vi "Queue_Driver.vi"(0 "Data_In":string, 1 "Max_Queue_Size (-1, unlimited)":i32=-1, 2 "Queue_Name":string, 5 "Data_In_N":string[](array[string]), 7 "Timeout (-1)":i32, 11 "Error_In":errorcluster, 13 "Queue_Operation_Select":T1=enum."Release_Queue") -> (4 "Data_Out":string, 15 "Error_Out":errorcluster)   [LabVIEW 2021]
doc: "This is the queue driver vi that creates, enqueues, dequeues and releases the queue."
uses:
  Control/Queue_Operation_Select.ctl
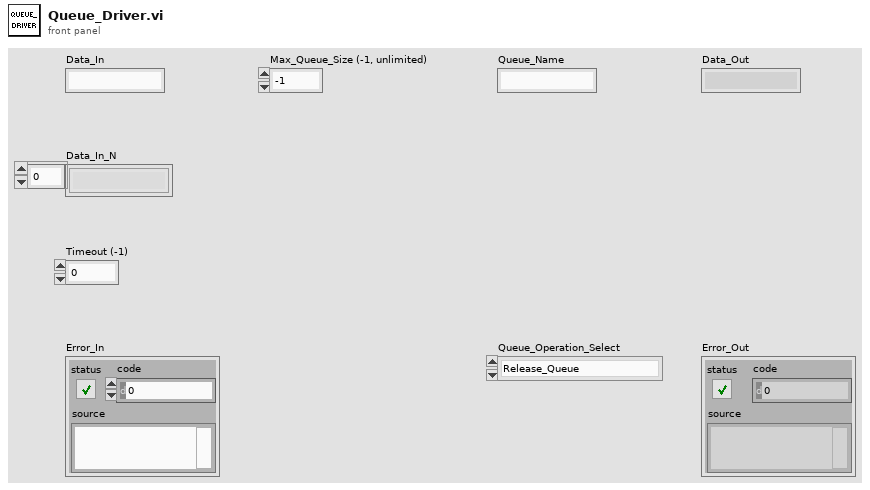
[diagram p1: front panel]
types:
  T1 = typedef "Queue_Operation_Select.ctl" = enum16{"Obtain_Queue", "Enqueue", "Enqueue_N", "Enqueue_at_First", "Dequeue", "Flush_Queue", "Release_Queue"}
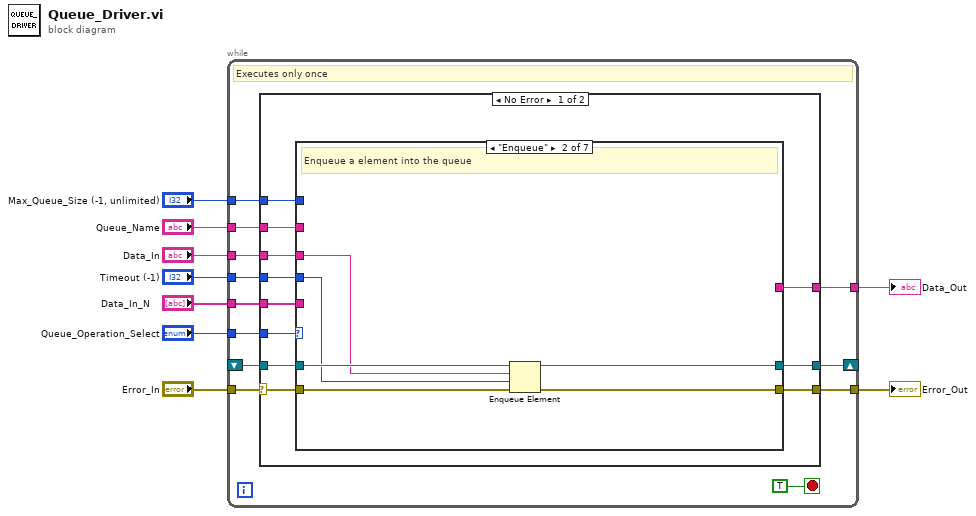
[diagram p0: block diagram]
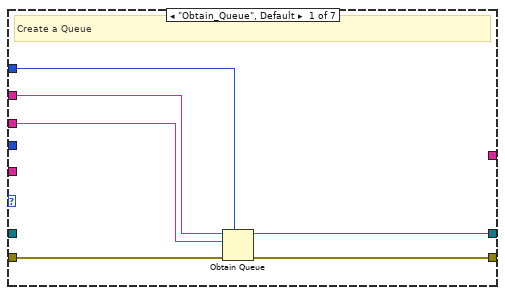
[diagram p2: hidden frame]
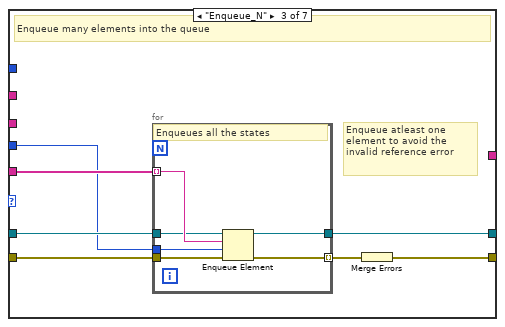
[diagram p3: hidden frame]
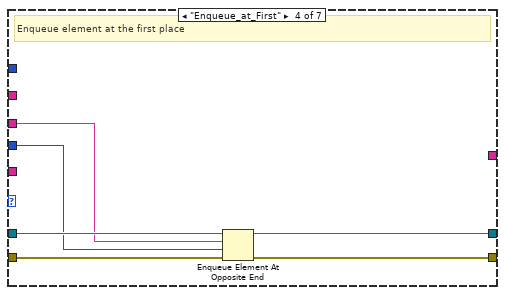
[diagram p4: hidden frame]
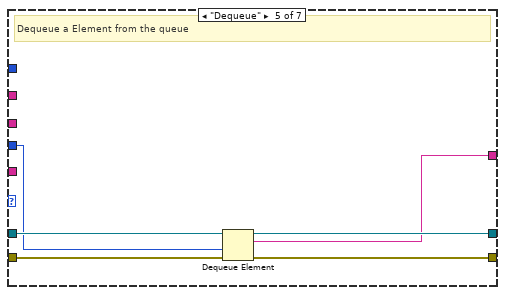
[diagram p5: hidden frame]
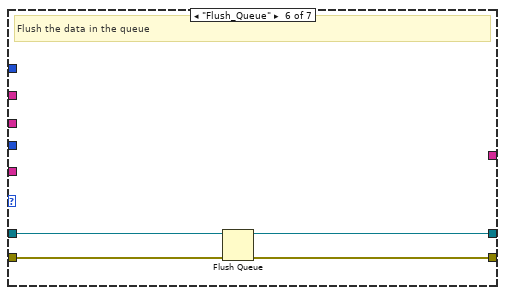
[diagram p6: hidden frame]
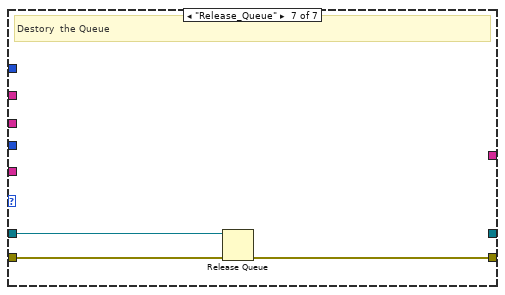
[diagram p7: hidden frame]
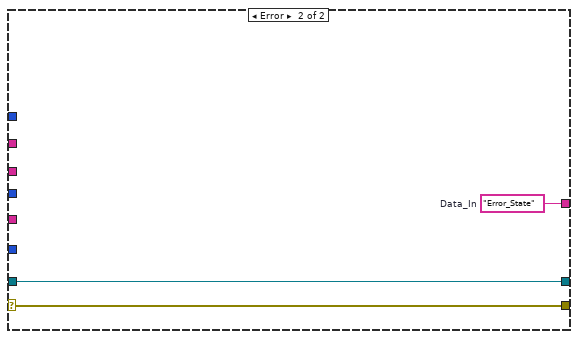
[diagram p8: hidden frame]
diagram:
  n1 = while {
    tunnel: "Error_In" -> [w21]
    tunnel: [w20] -> w8
    tunnel: "Queue_Operation_Select" -> [w19]
    tunnel: "Queue_Name" -> [w18]
    tunnel: "Data_In" -> [w17]
    tunnel: "Max_Queue_Size (-1, unlimited)" -> [w16]
    shift-right: [w15] -> _
    shift-left: _ -> [w14]
    tunnel: "Timeout (-1)" -> [w13]
    tunnel: "Data_In_N" -> [w12]
    tunnel: [w11] -> w1
    stop <- TRUE stop-if-true
    # "Executes only once"
    n2 = case shown="No Error" w21 {
      selector: w21 -> [w32 w78]
      tunnel: [w31 w78] -> w20
      tunnel: w19 -> [w30 _]
      tunnel: w18 -> [w29 _]
      tunnel: w17 -> [w28 _]
      tunnel: w16 -> [w27 _]
      tunnel: [w26 w79] -> w15
      tunnel: w14 -> [w25 w79]
      tunnel: w13 -> [w24 _]
      tunnel: w12 -> [w23 _]
      tunnel: [w22 w77] -> w11
      frame No Error {
        n3 = case shown="\"Enqueue\"" w30 {
          tunnel: w32 -> [w38 w44 w51 w63 w69 w73 w76]
          tunnel: [w37 w43 w46 w62 w68 w72 w75] -> w31
          tunnel: w29 -> [w36 _ _ _ _ _ _]
          tunnel: w28 -> [w35 w41 _ w60 _ _ _]
          tunnel: w27 -> [w34 _ _ _ _ _ _]
          tunnel: [w33 w39 w47 w58 w65 w70 _] -> w26
          tunnel: w25 -> [_ w42 w48 w61 w67 w71 w74]
          tunnel: w24 -> [_ w40 w45 w59 w66 _ _]
          tunnel: w23 -> [_ _ w49 _ _ _ _]
          tunnel: [_ _ _ _ w64 _ _] -> w22
          frame "Obtain_Queue", Default {
            # "Create a Queue"
            n4 = Obtain Queue(max queue size (-1, unlimited)=w34, name (unnamed)=w36, element data type=w35, error in (no error)=w38) -> (queue out=w33:refnum<queue>, error out=w37:errorcluster)  [unwired: 1 in, 1 out]
          }
          frame "Enqueue" {
            # "Enqueue a element into the queue"
            n5 = Enqueue Element(queue=w42, element=w41, timeout in ms (-1)=w40, error in (no error)=w44) -> (queue out=w39:refnum<queue>, error out=w43:errorcluster)  [unwired: 1 out]
          }
          frame "Enqueue_N" {
            # "Enqueue atleast one element to avoid the invalid reference error"
            # "Enqueue many elements into the queue"
            n6 = for {
              tunnel: w49 -> [w55] mode=indexing
              tunnel: w48 -> [w54]
              tunnel: [w53] -> w47
              tunnel: w51 -> [w57]
              tunnel: [w56] -> w50 mode=indexing
              tunnel: w45 -> [w52]
              # "Enqueues all the states"
              n7 = Enqueue Element(queue=w54, element=w55, timeout in ms (-1)=w52, error in (no error)=w57) -> (queue out=w53:refnum<queue>, error out=w56:errorcluster)  [unwired: 1 out]
            }
            n8 = Merge Errors(w50) -> (w46:errorcluster)
          }
          frame "Enqueue_at_First" {
            # "Enqueue element at the first place"
            n9 = Enqueue Element At Opposite End(queue=w61, element=w60, timeout in ms (-1)=w59, error in (no error)=w63) -> (queue out=w58:refnum<queue>, error out=w62:errorcluster)  [unwired: 1 out]
          }
          frame "Dequeue" {
            # "Dequeue a Element from the queue"
            n10 = Dequeue Element(queue=w67, timeout in ms (-1)=w66, error in (no error)=w69) -> (queue out=w65:refnum<queue>, element=w64:string, error out=w68:errorcluster)  [unwired: 1 out]
          }
          frame "Flush_Queue" {
            # "Flush the data in the queue"
            n11 = Flush Queue(queue=w71, error in (no error)=w73) -> (queue out=w70:refnum<queue>, error out=w72:errorcluster)  [unwired: 1 out]
          }
          frame "Release_Queue" {
            # "Destory  the Queue"
            n12 = Release Queue(queue=w74, error in (no error)=w76) -> (error out=w75:errorcluster)  [unwired: 1 in, 2 out]
          }
        }
      }
      frame Error {
        w77 = "Error_State"  # Data_In
      }
    }
  }
  "Error_Out" <- w8
  "Data_Out" <- w1
